vi "FTW-SEQ-Flush.vi"(3 "FTW Job Sequencer":refnum<class "FTW-JobSequencer.lvclass">) -> (0 "FTW Job Sequencer out":refnum<class "FTW-JobSequencer.lvclass">)   [LabVIEW 2015, in "FTW-JobSequencer.lvclass"]
uses:
  FTW-JobSequencer.lvclass
  FTW-JobSequencer.lvclass/FTW-JobSequencer.ctl
panel:
  # "Inputs"
  # "Outputs"
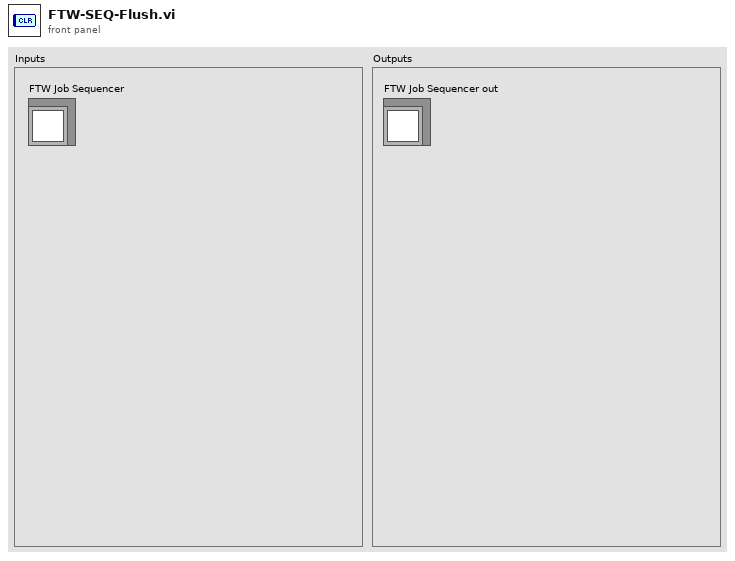
[diagram p1: front panel]
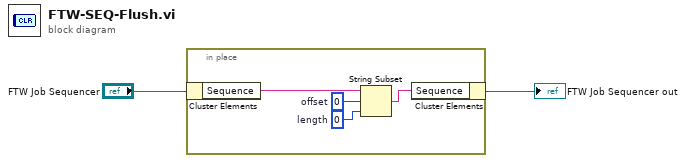
[diagram p0: block diagram]
diagram:
  n1 = in-place {
    w3 = 0  # offset
    w4 = 0  # length
    n2 = in-place-cluster #1("FTW Job Sequencer") -> ("Sequence"=w6:string)
    n3 = String Subset(string=w6, offset (0)=w3, length (rest)=w4) -> (substring=w5:string)
    n4 = in-place-cluster #1("Sequence"=w5) -> (→"FTW Job Sequencer out":refnum<class "FTW-JobSequencer.lvclass">)
  }
